vi "运维调试_采配水.vi"() -> ()   [LabVIEW 2016, in "PLC.lvlib"]
uses:
  PLC.lvlib
  <vilib>/Plasmionique/MB Master/MB_Master/MB_Master.lvclass
  <vilib>/Utility/miscctls.llb/LVPointTypeDef.ctl
  <vilib>/Plasmionique/MB Master/MB_Master_Serial/MB_Master_Serial.lvclass
  D:/Program Files (x86)/National Instruments/LabVIEW 2016/vi.lib/Plasmionique/MB Master/MB_Master/MB_Master.lvclass
  <vilib>/Plasmionique/MB Master/MB Master.lvlib
panel:
  out "Y7":bool caption="V6 空压机"
  out "Y6":bool caption="V5 排液阀"
  out "Y5":bool caption="V4 二级清洗阀"
  out "Y4":bool caption="V3 一级清洗阀"
  out "Y3":bool caption="V2 外部管路清洗阀"
  out "Y2":bool caption="M2 增压泵"
  out "Y1":bool caption="V1 进样阀"
  out "Y0":bool caption="M1 潜水泵"
  out "X7":bool caption="采水泵过载检测"
  out "X6":bool caption="断电检测"
  out "X5":bool caption="开门检测"
  out "X4":bool caption="烟雾检测"
  out "X3":bool caption="漏水检测"
  out "X2":bool caption="进样检测"
  out "X1":bool
  out "X0":bool caption="采样池液位开关"
  out "R109":i16 caption="配水时间"
  out "集成报警信息":string
  out "R108":i16 caption="自来水报警"
  out "R107":i16 caption="采水池液位报警设置"
  out "R106":i16 caption="进样超时设置"
  out "R105":i16 caption="二级清洗时间"
  out "R104":i16 caption="一级清洗时间"
  out "R103":i16 caption="外部管路清洗时间"
  out "R102":i16 caption="静置沉淀时间"
  out "R101":i16 caption="内部管路润洗时间"
  out "R100":i16 caption="外部管路润洗时间"
  out "R2":i16
  out "R1":i16
  out "多列列表框":i32(listbox)
  out "R19":i16
  out "R18":i16
  out "R17":i16
  out "R16":i16
  out "R15":i16
  out "R14":i16
  out "R13":i16
  out "R12":i16
  in  "V6":bool
  in  "V5":bool
  in  "V4":bool
  in  "V3":bool
  in  "V2":bool
  in  "M2":bool
  in  "V1":bool
  in  "M1":bool
  in  "返回":bool
  in  "参数设置":bool
  in  "单步启动":bool
  in  "启动":bool
  in  "停止":bool
  # "S"
  # "S"
  # "S"
  # "S"
  # "S"
  # "S"
  # "S"
  # "S"
  # "S"
  # "S"
  # "单步计时："
  # "s"
  # "流程计时："
  # "s"
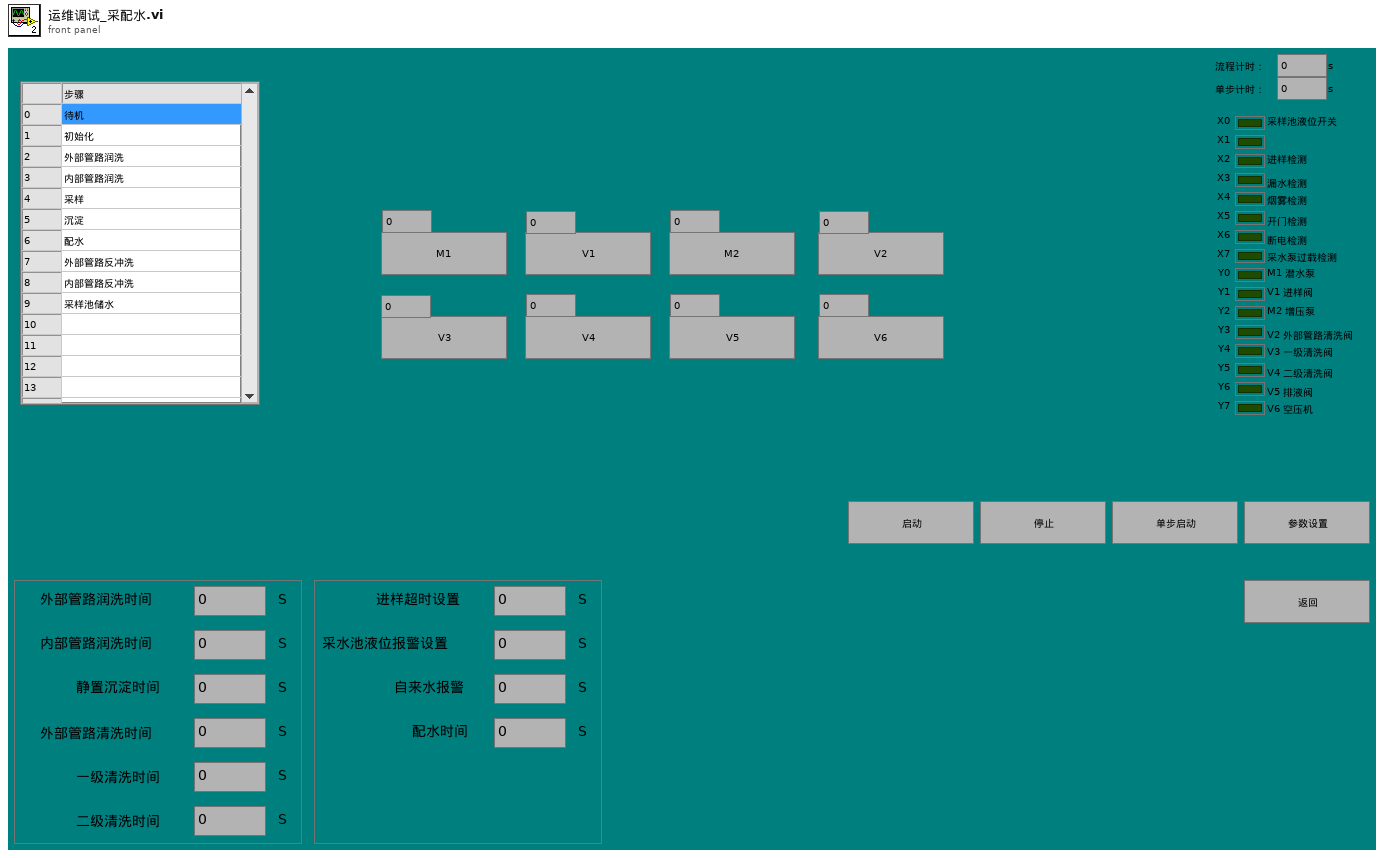
[diagram p1: front panel]
types:
  T1 = typedef "LVPointTypeDef.ctl" = cluster{"Horizontal":i16, "Vertical":i16}
  T2 = cluster{"时间标识":timestamp, "设备":string, "日志信息":string}
  T3 = cluster{"R0":i16, "R1":i16, "R2":i16, "R3":i16, "R4":i16, "R5":i16, "R6":i16, "R7":i16, "R8":i16, "R9":i16, "R10":i16, "R11":i16, "R12":i16, "R13":i16, "R14":i16, "R15":i16, "R16":i16, "R17":i16, "R18":i16, "R19":i16}
  T4 = cluster{"coil values[0]":bool, "coil values[1]":bool, "coil values[2]":bool, "coil values[3]":bool, "coil values[4]":bool, "coil values[5]":bool, "coil values[6]":bool, "coil values[7]":bool, "coil values[8]":bool, "coil values[9]":bool, "coil values[10]":bool, "coil values[11]":bool, "coil values[12]":bool, "coil values[13]":bool, "coil values[14]":bool, "coil values[15]":bool}
  T5 = cluster{"seconds since 1Jan1904":timestamp, "table输入":string, string, "table输入":string}
  T6 = cluster{"时间标识":timestamp, "设备":string, "日志信息":string, "流程参数":string}
  T7 = cluster{"命令":string, cluster{"starting address":u16, "holding register value":u16}}
  T8 = cluster{"命令":string, "数据":cluster{"starting address":u16, "holding register value":u16}}
  T9 = cluster{"命令":string, "数据":cluster{"starting address":u16, "holding register values":u16[]}}
  T10 = cluster{"命令":string, "data":cluster{"starting address":u16, "coil values":bool[]}}
  T11 = enum32{"Bad", "Idle", "Run top level", "Running"}
  T12 = cluster{"baud rate (bps)":u32, "stop bits":u16, "parity":u16, "flow control":u16, "timeout":u32, "retries":i32}
  T13 = cluster{"starting address":u16, "holding register values":u16[]}
  T14 = cluster{"starting address":u16, "holding register value":u16}
  T15 = cluster{"starting address":u16, "coil values":bool[]}
  T16 = cluster{"Registers[0]":u16, "Registers[1]":u16, "Registers[2]":u16, "Registers[3]":u16, "Registers[4]":u16, "Registers[5]":u16, "Registers[6]":u16, "Registers[7]":u16, "Registers[8]":u16, "Registers[9]":u16, "Registers[10]":u16, "Registers[11]":u16, "Registers[12]":u16, "Registers[13]":u16, "Registers[14]":u16, "Registers[15]":u16, "Registers[16]":u16, "Registers[17]":u16, "Registers[18]":u16, "Registers[19]":u16}
  T17 = cluster{"Registers[0]":u16, "Registers[1]":u16, "Registers[2]":u16, "Registers[3]":u16, "Registers[4]":u16, "Registers[5]":u16}
  T18 = cluster{"Coils[0]":bool, "Coils[1]":bool, "Coils[2]":bool, "Coils[3]":bool, "Coils[4]":bool, "Coils[5]":bool, "Coils[6]":bool, "Coils[7]":bool, "Coils[8]":bool, "Coils[9]":bool, "Coils[10]":bool, "Coils[11]":bool, "Coils[12]":bool, "Coils[13]":bool, "Coils[14]":bool, "Coils[15]":bool}
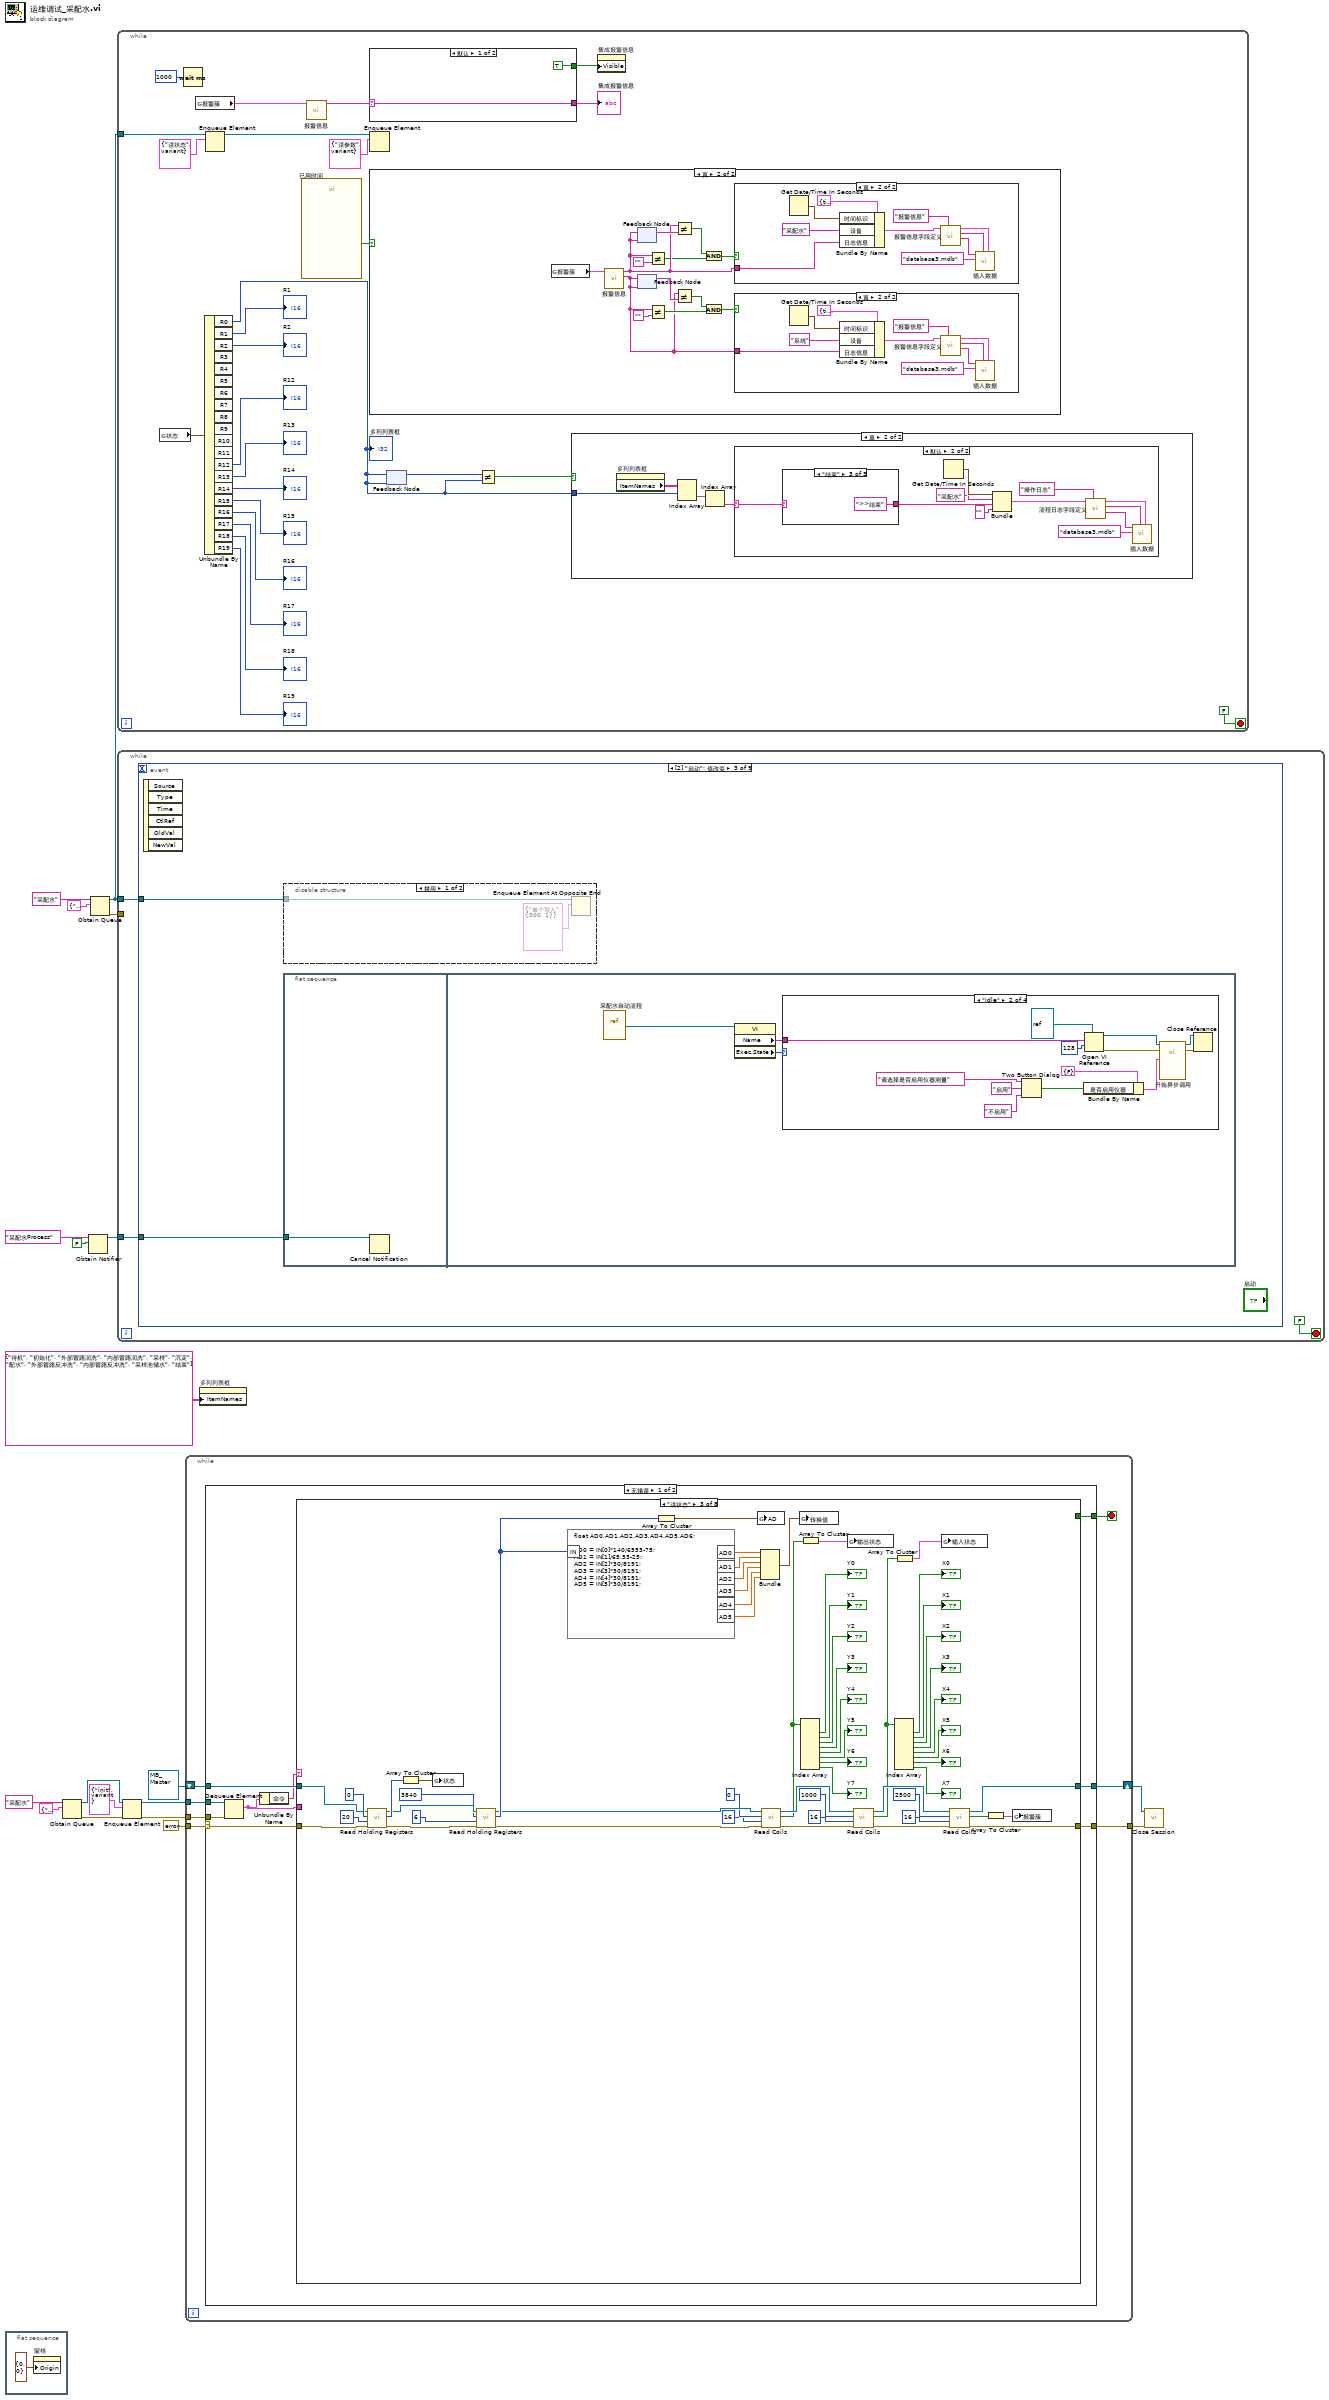
[diagram p0: block diagram]
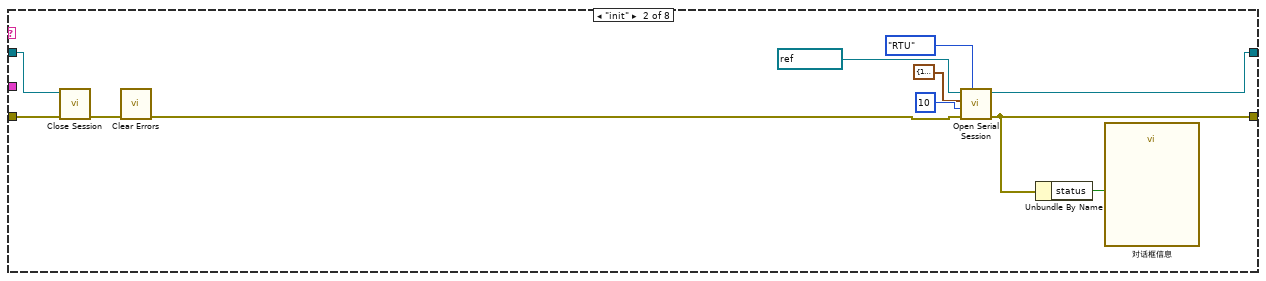
[diagram p3: hidden frame]
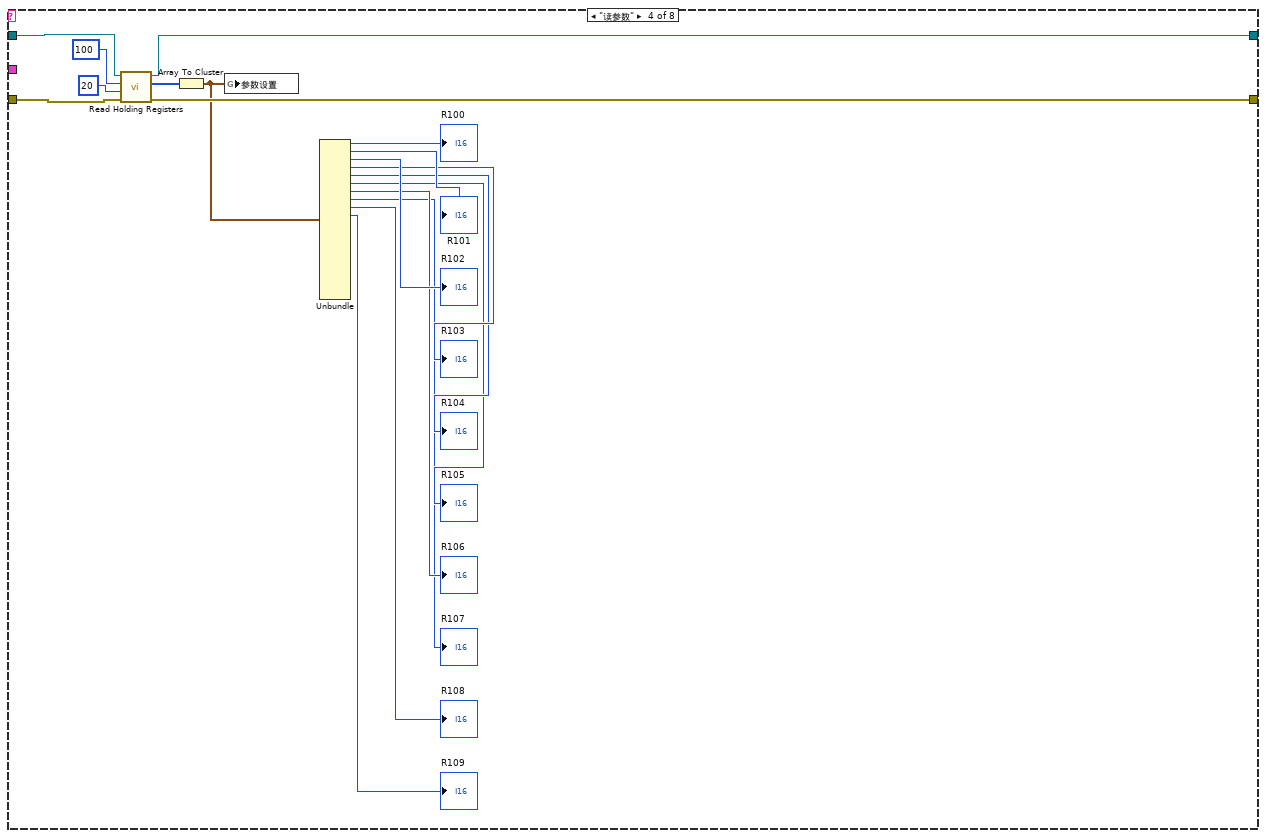
[diagram p4: hidden frame]
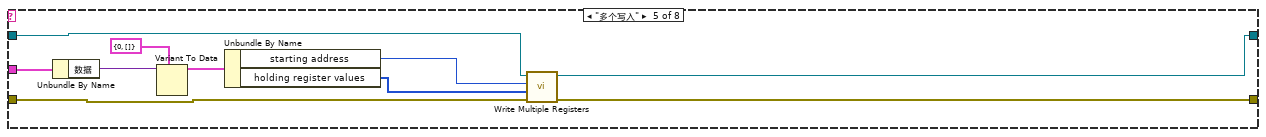
[diagram p5: hidden frame]
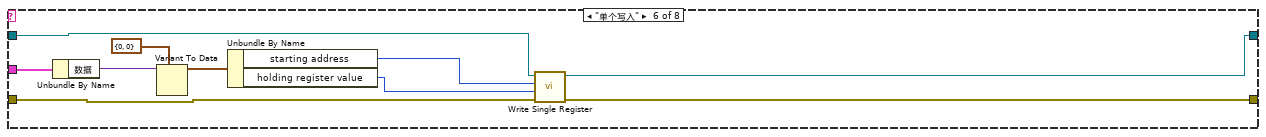
[diagram p6: hidden frame]
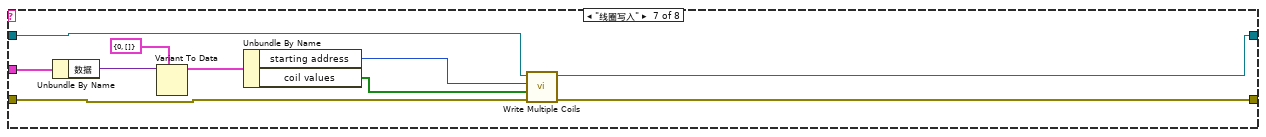
[diagram p7: hidden frame]
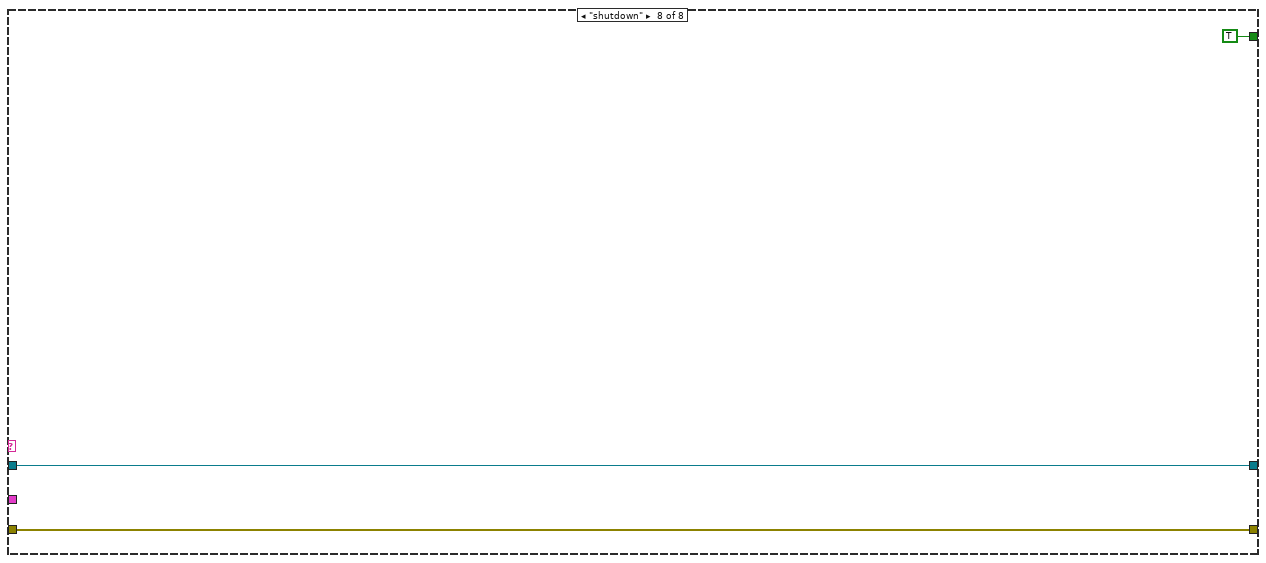
[diagram p8: hidden frame]
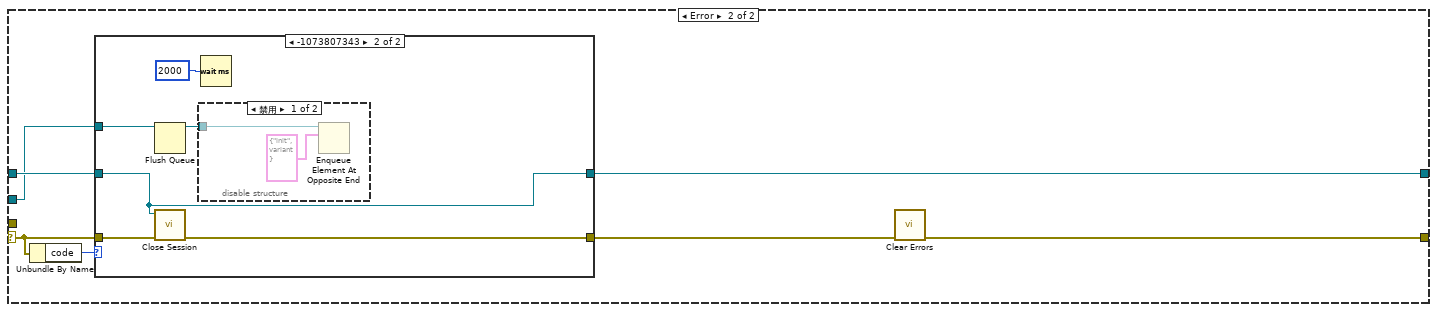
[diagram p9: hidden frame]
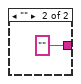
[diagram p15: hidden frame]
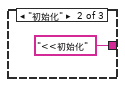
[diagram p19: hidden frame]
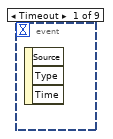
[diagram p20: hidden frame]
diagram:
  n1 = flat-sequence {
    frame #0 {
      n2 = property on="窗格" class="Pane"("Origin"=T1 {"Horizontal"=0, "Vertical"=0} ("原点")) -> ()  [unwired: 2 in, 2 out]
    }
  }
  n3 = Obtain Queue(name (unnamed)="采配水" ("名称（未命名）"), element data type=cluster{"命令":string, "数据":variant} {"命令"="", "数据"=variant}) -> (queue out=w9:refnum<queue>, error out=w8:errorcluster)  [unwired: 3 in, 1 out]
  n4 = Obtain Notifier(name (unnamed)="采配水Process" ("名称（未命名）"), notification data type=FALSE) -> (notifier out=w12:refnum<notifier>)  [unwired: 2 in, 2 out]
  n5 = Obtain Queue(name (unnamed)="采配水" ("名称（未命名）"), element data type=cluster{"命令":string, "数据":variant} {"命令"="", "数据"=variant}) -> (queue out=w16:refnum<queue>, error out=w17:errorcluster)  [unwired: 3 in, 1 out]
  n6 = while {
    tunnel: w16 -> [w44]
    stop <- FALSE stop-if-true
    n7 = global read "采配水全局变量.vi" "状态"() -> (w42:T3)
    n8 = Wait (ms)(milliseconds to wait=u32 1000 ("等待时间（毫秒）")) -> ()  [unwired: 1 out]
    n9 = global read "采配水全局变量.vi" "报警簇"() -> (w30:T4)
    n10 = Unbundle By Name(w42) -> ("R0"=w21:i16, "R1"=→"R1":i16, "R2"=→"R2":i16, "R12"=→"R12":i16, "R13"=→"R13":i16, "R14"=→"R14":i16, "R15"=→"R15":i16, "R16"=→"R16":i16, "R17"=→"R17":i16, "R18"=→"R18":i16, "R19"=→"R19":i16)  [unwired: 9 out]
    "多列列表框" <- w21
    n11 = Enqueue Element(queue=w44, element=cluster{"命令":string, "数据":variant} {"命令"="读状态", "数据"=variant} ("元素")) -> (queue out=w24:refnum<queue>)  [unwired: 2 in, 2 out]
    n12 = call "已用时间"() -> ("Time has Elapsed"=w27:bool)  [unwired: 12 in, 7 out]
    n13 = call "报警信息.vi"("报警簇"=w30) -> ("采配水报警信息"=w23:string)  [unwired: 9 in, 1 out]
    n14 = case shown="默认" w23 {
      selector: w23 -> [w80 _]
      tunnel: [w80 "" ("字符串")] -> w29
      tunnel: [TRUE ("可见") _] -> w28
      frame Default {
      }
      frame "" {
      }
    }
    "集成报警信息" <- w29
    n15 = Enqueue Element(queue=w24, element=cluster{"命令":string, "数据":variant} {"命令"="读参数", "数据"=variant} ("元素")) -> ()  [unwired: 2 in, 3 out]
    n16 = case shown="真" w27 {
      frame False {
      }
      frame True {
        n17 = global read "采配水全局变量.vi" "报警簇"() -> (w58:T4)
        n18 = call "报警信息.vi"("报警簇"=w58) -> ("系统报警信息"=w47:string, "采配水报警信息"=w54:string)  [unwired: 9 in]
        n19 = feedback #1(w54) -> (w57:string)
        n20 = feedback-in #1(w54) -> ()
        n21 = feedback #2(w47) -> (w48:string)
        n22 = feedback-in #2(w47) -> ()
        n23 = Not Equal?(x=w54, y="") -> (x != y?=w52:bool)
        n24 = Not Equal?(x=w47, y="") -> (x != y?=w51:bool)
        n25 = Not Equal?(x=w54, y=w57) -> (x != y?=w56:bool)
        n26 = Not Equal?(x=w47, y=w48) -> (x != y?=w49:bool)
        n27 = And(x=w56, y=w52) -> (x .and. y?=w55:bool)
        n28 = And(x=w49, y=w51) -> (x .and. y?=w46:bool)
        n29 = case shown="真" w55 {
          tunnel: w54 -> [_ w69]
          frame False {
          }
          frame True {
            n30 = Get Date/Time In Seconds() -> (seconds since 1Jan1904=w71:timestamp)
            n31 = Bundle By Name(cluster=T2 {"时间标识"=timestamp(0 s since 1904-01-01), "设备"="", "日志信息"=""} ("data in"), "时间标识"=w71, "设备"="采配水", "日志信息"=w69) -> (w72:T2)
            n32 = call "报警信息字段定义.vi"("table输入"="报警信息", "data in"=w72) -> ("table输出"=w76:string, "columns"=w77:string[], "data out"=w78:T2)  [unwired: 7 in]
            n33 = call "插入数据.vi"("data"=w78, "columns"=w77, "database"="database3.mdb", "table"=w76) -> ()  [unwired: 7 in, 1 out]
          }
        }
        n34 = case shown="真" w46 {
          tunnel: w47 -> [_ w59]
          frame False {
          }
          frame True {
            n35 = Get Date/Time In Seconds() -> (seconds since 1Jan1904=w61:timestamp)
            n36 = Bundle By Name(cluster=T2 {"时间标识"=timestamp(0 s since 1904-01-01), "设备"="", "日志信息"=""} ("data in"), "时间标识"=w61, "设备"="系统", "日志信息"=w59) -> (w62:T2)
            n37 = call "报警信息字段定义.vi"("table输入"="报警信息", "data in"=w62) -> ("table输出"=w66:string, "columns"=w67:string[], "data out"=w68:T2)  [unwired: 7 in]
            n38 = call "插入数据.vi"("data"=w68, "columns"=w67, "database"="database3.mdb", "table"=w66) -> ()  [unwired: 7 in, 1 out]
          }
        }
      }
    }
    n39 = feedback-in #3(w21) -> ()
    n40 = feedback #3(w21) -> (w22:i16)
    n41 = Not Equal?(x=w22, y=w21) -> (x != y?=w31:bool)
    n42 = case shown="真" w31 {
      tunnel: w21 -> [_ w84]
      frame False {
      }
      frame True {
        n43 = property on="多列列表框" class="MCListbox (严格)"() -> ("ItemNames"=w85:string[][])  [unwired: 2 in, 2 out]
        n44 = Index Array(array=w85, index (row)=w84) -> (element=w83:string[])  [unwired: 1 in]
        n45 = Index Array(array=w83) -> (element=w82:string)  [unwired: 1 in]
        n46 = case shown="默认" w82 {
          selector: w82 -> [_ w87]
          frame "待机" {
          }
          frame Default {
            n47 = case shown="\"结束\"" w87 {
              selector: w87 -> [w97 _ _]
              tunnel: [w97 "<<初始化" ">>结束"] -> w86
              frame Default {
              }
              frame "初始化" {
              }
              frame "结束" {
              }
            }
            n48 = Get Date/Time In Seconds() -> (seconds since 1Jan1904=w91:timestamp)
            n49 = Bundle("seconds since 1Jan1904"=w91, "table输入"="采配水", w86, "table输入"="") -> (w89:T5)  [unwired: 1 in]
            n50 = call "流程日志字段定义.vi"("table输入"="操作日志", "data in"=w89) -> ("table输出"=w94:string, "columns"=w95:string[], "data out"=w96:T6)  [unwired: 7 in]
            n51 = call "插入数据.vi"("data"=w96, "columns"=w95, "database"="database3.mdb", "table"=w94) -> ()  [unwired: 7 in, 1 out]
          }
        }
      }
    }
    n52 = property on="集成报警信息" class="Str"("Visible"=w28) -> ()  [unwired: 2 in, 2 out]
  }
  n53 = while {
    tunnel: w16 -> [w101]
    tunnel: w17 -> [_]
    tunnel: w12 -> [w100]
    stop <- FALSE stop-if-true
    n54 = event shown="[2] \"启动\": 值改变" {
      selector: _ -> [_ _ _ _ _ _ _ _ _]
      dyn-events: _ -> [_ _ _ _ _ _ _ _ _]
      timeout: _ -> [_ _ _ _ _ _ _ _ _]
      tunnel: w101 -> [_ w105 w108 w132 w147 _ _ _ w165]
      tunnel: w100 -> [_ w104 w107 _ _ _ _ _ _]
      event Timeout {
        n55 = event-data() -> ()  [unwired: 1 in, 3 out]
      }
      event "停止": Value Change {
        n56 = event-data() -> ()  [unwired: 1 in, 6 out]
        n57 = Send Notification(notification=TRUE ("通知"), notifier=w104) -> ()  [unwired: 1 in, 2 out]
        n58 = Enqueue Element At Opposite End(queue=w105, element=T7 {"命令"="单个写入", {"starting address"=300, "holding register value"=2}} ("元素")) -> ()  [unwired: 2 in, 3 out]
      }
      event "启动": Value Change {
        n59 = event-data() -> ()  [unwired: 1 in, 6 out]
        n60 = disable-structure shown="禁用" {
          disable-tunnel: w108 -> [w128 _]
          frame Disabled {
            n61 = Enqueue Element At Opposite End(queue=w128, element=T7 {"命令"="单个写入", {"starting address"=300, "holding register value"=1}} ("元素")) -> ()  [unwired: 2 in, 3 out]
          }
          frame Enabled {
          }
        }
        n62 = flat-sequence {
          tunnel: w107 -> [w109]
          frame #0 {
            n63 = Cancel Notification(0:w109) -> ()  [unwired: 1 in, 3 out]
          }
          frame #1 {
            n64 = vi-ref "采配水自动流程.vi"() -> (w112:refnum<vi>)
            n65 = property class="VI"(reference=w112) -> ("Name"=w111:string, "Exec.State"=w110:T11)  [unwired: 1 in, 2 out]
            n66 = case shown="\"Idle\"" w110 {
              tunnel: w111 -> [_ w125 _ _]
              frame "Bad", Default {
              }
              frame "Idle" {
                n67 = Two Button Dialog(message="请选择是否启用仪器测量" ("消息"), 1:"不启用" ("F按钮名称（“取消”）"), 2:"启用" ("T按钮名称（“确定”）")) -> (T button?=w115:bool)
                n68 = Bundle By Name(cluster=cluster{"是否启用仪器":bool} {"是否启用仪器"=FALSE} ("参数"), "是否启用仪器"=w115) -> (w113:cluster{"是否启用仪器":bool})
                n69 = Open VI Reference(type specifier VI Refnum (for type only)=refnum<vi> refnum, vi path=w125, options=128 ("选项")) -> (vi reference=w123:refnum<vi>, error out=w120:errorcluster)  [unwired: 3 in]
                n70 = call-by-ref "开始异步调用"(reference=w123, error in=w120, "参数"=w113) -> (reference out=w121:refnum<vi>, error out=w119:errorcluster)  [unwired: 11 in]
                n71 = Close Reference(reference=w121, error in (no error)=w119) -> ()  [unwired: 1 out]
              }
              frame "Run top level" {
              }
              frame "Running" {
                n72 = One Button Dialog(message="流程已经运行,无须重复启动" ("消息")) -> ()  [unwired: 1 in, 1 out]
              }
            }
          }
        }
      }
      event "单步启动": Value Change {
        n73 = event-data() -> ()  [unwired: 1 in, 6 out]
        n74 = call "单步启动对话框.vi"() -> ("单步启动步骤输出"=w129:u16)  [unwired: 11 in]
        n75 = Bundle By Name(cluster=T8 {"命令"="单个写入", "数据"={"starting address"=301, "holding register value"=0}} ("元素"), "数据.holding register value"=w129) -> (w130:T8)
        n76 = Enqueue Element At Opposite End(queue=w132, element=w130) -> ()  [unwired: 2 in, 3 out]
      }
      event "R100", "R101", "R102", "R103", "R104", "R105", "R106", "R107", "R108", "R109": Value Change {
        n77 = event-data() -> ()  [unwired: 1 in, 6 out]
        n78 = local read "R100"() -> (w142:i16)
        n79 = local read "R101"() -> (w141:i16)
        n80 = local read "R102"() -> (w140:i16)
        n81 = local read "R103"() -> (w139:i16)
        n82 = local read "R104"() -> (w138:i16)
        n83 = local read "R105"() -> (w137:i16)
        n84 = local read "R106"() -> (w136:i16)
        n85 = local read "R107"() -> (w135:i16)
        n86 = local read "R108"() -> (w134:i16)
        n87 = local read "R109"() -> (w133:i16)
        n88 = Build Array(w142, w141, w140, w139, w138, w137, w136, w135, w134, w133) -> (w143:i16[])
        n89 = Bundle By Name(cluster=T9 {"命令"="多个写入", "数据"={"starting address"=0, "holding register values"=[]}} ("元素"), "数据.starting address"=u16 100, "数据.holding register values"=w143) -> (w144:T9)
        n90 = Enqueue Element At Opposite End(queue=w147, element=w144) -> ()  [unwired: 2 in, 3 out]
      }
      event "R100", "R101", "R102", "R103", "R104", "R105", "R106", "R107", "R108", "R109": Mouse Down {
        n91 = event-data() -> ("CtlRef"=w151:refnum<vi>)  [unwired: 1 in, 7 out]
        n92 = property class="DigNum (严格)"(reference=w151) -> (reference out=w149:refnum<vi>, "Value"=w150:i16)  [unwired: 1 in, 1 out]
        n93 = call "数字键盘.vi"("OldNumber"=w150) -> ("NewNumber"=w148:sgl)
        n94 = property class="DigNum (严格)"(reference=w149, "Val(Sgnl)"=w148) -> ()  [unwired: 1 in, 2 out]
      }
      event "参数设置": Value Change {
        n95 = event-data() -> ()  [unwired: 1 in, 6 out]
        n96 = property on="窗格" class="Pane"("Origin"=T1 {"Horizontal"=0, "Vertical"=528} ("原点")) -> ()  [unwired: 2 in, 2 out]
      }
      event "返回": Value Change {
        n97 = event-data() -> ()  [unwired: 1 in, 6 out]
        n98 = property on="窗格" class="Pane"("Origin"=T1 {"Horizontal"=0, "Vertical"=0} ("原点")) -> ()  [unwired: 2 in, 2 out]
      }
      event "M1", "V1", "M2", "V2", "V3", "V4", "V5", "V6": Value Change {
        n99 = event-data() -> ()  [unwired: 1 in, 6 out]
        n100 = Build Array("M1", "V1", "M2", "V2", "V3", "V4", "V5", "V6") -> (w154:bool[])
        n101 = Bundle By Name(cluster=T10 {"命令"="线圈写入", "data"={"starting address"=2400, "coil values"=[]}} ("元素"), "data.coil values"=w154) -> (w155:T10)
        n102 = Enqueue Element(queue=w165, element=w155) -> ()  [unwired: 2 in, 3 out]
      }
    }
  }
  n103 = Enqueue Element(queue=w9, element=cluster{"命令":string, "数据":variant} {"命令"="init", "数据"=variant} ("元素"), error in (no error)=w8) -> (queue out=w4:refnum<queue>, error out=w6:errorcluster)  [unwired: 1 in, 1 out]
  n104 = while {
    tunnel: w4 -> [w168]
    tunnel: w6 -> [w167]
    shift-right: [w172] -> w1
    shift-left: refnum<class "MB_Master.lvclass"> refnum ("MB session in") -> [w171]
    tunnel: errorcluster {"status"=FALSE, "code"=0, "source"=""} ("error out") -> [w169]
    tunnel: [w170] -> w2
    stop <- w166 stop-if-true
    n105 = case shown="无错误" w169 {
      selector: w169 -> [w178 w305]
      tunnel: [w181 w304] -> w172
      tunnel: w171 -> [w180 w306]
      tunnel: [w179 w302] -> w170
      tunnel: w168 -> [w175 w301]
      tunnel: w167 -> [w174 _]
      tunnel: [w176 _] -> w166
      frame No Error {
        n106 = Dequeue Element(queue=w175, error in (no error)=w174) -> (element=w173:cluster{"命令":string, "数据":variant})  [unwired: 1 in, 3 out]
        n107 = Unbundle By Name(w173) -> ("命令"=w177:string)
        n108 = case shown="\"读状态\"" w177 {
          tunnel: [w183 w187 w214 w262 w274 w284 w294 w299] -> w181
          tunnel: w180 -> [w183 w191 w234 w267 w277 w287 w297 w299]
          tunnel: [w182 w189 w213 w261 w275 w285 w295 w298] -> w179
          tunnel: w178 -> [w182 w193 w237 w266 w276 w286 w296 w298]
          tunnel: [_ _ _ _ _ _ _ TRUE] -> w176
          tunnel: w173 -> [_ _ _ _ w273 w283 w293 _]
          frame "idle", Default {
          }
          frame "init" {
            n109 = call-dynamic "Close Session.vi"("error in (no error)"=w193, "MB session in"=w191) -> ("error out"=w192:errorcluster)  [unwired: 9 in]
            n110 = call <vilib>:"Clear Errors.vi"("error in (no error)"=w192) -> ("error out"=w190:errorcluster)  [unwired: 5 in, 1 out]
            n111 = call <vilib>:"Open Serial Session.vi"("Mode (RTU)"=enum16{"RTU", "ASCII"}."RTU", "Error in"=w190, "Slave ID"=u8 10, "Serial Config"=T12 {"baud rate (bps)"=115200, "stop bits"=10, "parity"=0, "flow control"=0, "timeout"=1000, "retries"=1}, "VISA Resource"=refnum<visa-resource-name> "COM2" ("VISA resource name")) -> ("Error out"=w189:errorcluster, "MB_Serial session"=w187:refnum<class "MB_Master_Serial.lvclass">)  [unwired: 5 in]
            n112 = Unbundle By Name(w189) -> ("status"=w194:bool)
            n113 = call "对话框信息"("Enable"=w194) -> ()  [unwired: 9 in, 2 out]
          }
          frame "读状态" {
            n114 = call <vilib>:"Read Holding Registers.vi"("error in (no error)"=w237, "quantity"=u16 20 ("number of holding registers"), "starting address"=u16 0, "MB session in"=w234) -> ("error out"=w230:errorcluster, "Registers"=w233:u16[], "MB session out"=w232:refnum<class "MB_Master.lvclass">)  [unwired: 5 in]
            n115 = Array To Cluster(array=w233) -> (cluster=w239:T16)
            n116 = global write "采配水全局变量.vi" "状态"(w239) -> ()
            n117 = call <vilib>:"Read Holding Registers.vi"("error in (no error)"=w230, "quantity"=u16 6 ("number of holding registers"), "starting address"=u16 3840, "MB session in"=w232) -> ("error out"=w226:errorcluster, "Registers"=w231:u16[], "MB session out"=w227:refnum<class "MB_Master.lvclass">)  [unwired: 5 in]
            n118 = formula code="float AD0,AD1,AD2,AD3,AD4,AD5,AD6;\n\nAD0 = IN[0]*140/6553-75;\nAD1 = IN[1]/65.53-25;\nAD2 = IN[2]*30/8191;\nAD3 = IN[3]*30/8191;\nAD4 = IN[4]*30/8191;\nAD5 = IN[5]*30/8191;"("IN"=w231) -> ("AD0"=w245:dbl, "AD1"=w244:dbl, "AD2"=w243:dbl, "AD3"=w242:dbl, "AD4"=w241:dbl, "AD5"=w240:dbl)
            n119 = Array To Cluster(array=w231) -> (cluster=w247:T17)
            n120 = global write "采配水全局变量.vi" "AD"(w247) -> ()
            n121 = Bundle(w245, w244, w243, w242, w241, w240) -> (w246:cluster{dbl, dbl, dbl, dbl, dbl, dbl})  [unwired: 1 in]
            n122 = call <vilib>:"Read Coils.vi"("error in (no error)"=w226, "quantity"=u16 16 ("number of coils"), "starting address"=u16 0, "MB session in"=w227) -> ("error out"=w222:errorcluster, "Coils"=w203:bool[], "MB session out"=w223:refnum<class "MB_Master.lvclass">)  [unwired: 5 in]
            n123 = global write "采配水全局变量.vi" "转换值"(w246) -> ()
            n124 = Index Array(array=w203) -> (element #1=→"Y0":bool, element #2=→"Y1":bool, element #3=→"Y2":bool, element #4=→"Y3":bool, element #5=→"Y4":bool, element #6=→"Y5":bool, element #7=→"Y6":bool, element #8=→"Y7":bool)  [unwired: 8 in]
            n125 = Array To Cluster(array=w203) -> (cluster=w248:T18)
            n126 = global write "采配水全局变量.vi" "输出状态"(w248) -> ()
            n127 = call <vilib>:"Read Coils.vi"("error in (no error)"=w222, "quantity"=u16 16 ("number of coils"), "starting address"=u16 1000, "MB session in"=w223) -> ("error out"=w218:errorcluster, "Coils"=w212:bool[], "MB session out"=w219:refnum<class "MB_Master.lvclass">)  [unwired: 5 in]
            n128 = Index Array(array=w212) -> (element #1=→"X0":bool, element #2=→"X1":bool, element #3=→"X2":bool, element #4=→"X3":bool, element #5=→"X4":bool, element #6=→"X5":bool, element #7=→"X6":bool, element #8=→"X7":bool)  [unwired: 8 in]
            n129 = Array To Cluster(array=w212) -> (cluster=w249:T18)
            n130 = global write "采配水全局变量.vi" "输入状态"(w249) -> ()
            n131 = call <vilib>:"Read Coils.vi"("error in (no error)"=w218, "quantity"=u16 16 ("number of coils"), "starting address"=u16 2500, "MB session in"=w219) -> ("error out"=w213:errorcluster, "Coils"=w215:bool[], "MB session out"=w214:refnum<class "MB_Master.lvclass">)  [unwired: 5 in]
            n132 = Array To Cluster(array=w215) -> (cluster=w238:T18)
            n133 = global write "采配水全局变量.vi" "报警簇"(w238) -> ()
          }
          frame "读参数" {
            n134 = call <vilib>:"Read Holding Registers.vi"("error in (no error)"=w266, "quantity"=u16 20 ("number of holding registers"), "starting address"=u16 100, "MB session in"=w267) -> ("error out"=w261:errorcluster, "Registers"=w263:u16[], "MB session out"=w262:refnum<class "MB_Master.lvclass">)  [unwired: 5 in]
            n135 = Array To Cluster(array=w263) -> (cluster=w250:T16)
            n136 = global write "采配水全局变量.vi" "参数设置"(w250) -> ()
            n137 = Unbundle(w250) -> ("Registers[0]"=→"R100":u16, "Registers[1]"=→"R101":u16, "Registers[2]"=→"R102":u16, "Registers[3]"=→"R103":u16, "Registers[4]"=→"R104":u16, "Registers[5]"=→"R105":u16, "Registers[6]"=→"R106":u16, "Registers[7]"=→"R107":u16, "Registers[8]"=→"R108":u16, "Registers[9]"=→"R109":u16)  [unwired: 10 out]
          }
          frame "多个写入" {
            n138 = Unbundle By Name(w273) -> ("数据"=w272:variant)
            n139 = Variant To Data(type=T13 {"starting address"=0, "holding register values"=[]}, Variant=w272) -> (data=w270:T13)  [unwired: 1 in, 1 out]
            n140 = Unbundle By Name(w270) -> ("starting address"=w269:u16, "holding register values"=w268:u16[])
            n141 = call <vilib>:"Write Multiple Registers.vi"("error in (no error)"=w276, "values"=w268, "starting address"=w269, "MB session in"=w277) -> ("error out"=w275:errorcluster, "MB session out"=w274:refnum<class "MB_Master.lvclass">)  [unwired: 6 in]
          }
          frame "单个写入" {
            n142 = Unbundle By Name(w283) -> ("数据"=w282:variant)
            n143 = Variant To Data(type=T14 {"starting address"=0, "holding register value"=0}, Variant=w282) -> (data=w280:T14)  [unwired: 1 in, 1 out]
            n144 = Unbundle By Name(w280) -> ("starting address"=w279:u16, "holding register value"=w278:u16)
            n145 = call <vilib>:"Write Single Register.vi"("error in (no error)"=w286, "value"=w278, "address"=w279, "MB session in"=w287) -> ("error out"=w285:errorcluster, "MB session out"=w284:refnum<class "MB_Master.lvclass">)  [unwired: 6 in]
          }
          frame "线圈写入" {
            n146 = Unbundle By Name(w293) -> ("数据"=w292:variant)
            n147 = Variant To Data(type=T15 {"starting address"=0, "coil values"=[]}, Variant=w292) -> (data=w290:T15)  [unwired: 1 in, 1 out]
            n148 = Unbundle By Name(w290) -> ("starting address"=w289:u16, "coil values"=w288:bool[])
            n149 = call <vilib>:"Write Multiple Coils.vi"("error in (no error)"=w296, "values"=w288, "starting address"=w289, "MB session in"=w297) -> ("error out"=w295:errorcluster, "MB session out"=w294:refnum<class "MB_Master.lvclass">)  [unwired: 6 in]
          }
          frame "shutdown" {
          }
        }
      }
      frame Error {
        n150 = Unbundle By Name(w305) -> ("code"=w307:i32)
        n151 = case shown="-1073807343" w307 {
          tunnel: w306 -> [w309 w313]
          tunnel: w305 -> [w308 w315]
          tunnel: [w308 w314] -> w303
          tunnel: [w309 w313] -> w304
          tunnel: w301 -> [_ w312]
          frame Default {
          }
          frame -1073807343 {
            n152 = Flush Queue(queue=w312) -> (queue out=w311:refnum<queue>)  [unwired: 1 in, 2 out]
            n153 = call-dynamic "Close Session.vi"("error in (no error)"=w315, "MB session in"=w313) -> ("error out"=w314:errorcluster)  [unwired: 9 in]
            n154 = disable-structure shown="禁用" {
              disable-tunnel: w311 -> [w316 _]
              frame Disabled {
                n155 = Enqueue Element At Opposite End(queue=w316, element=cluster{"命令":string, "数据":variant} {"命令"="init", "数据"=variant} ("元素")) -> ()  [unwired: 2 in, 3 out]
              }
              frame Enabled {
              }
            }
            n156 = Wait (ms)(milliseconds to wait=u32 2000 ("等待时间（毫秒）")) -> ()  [unwired: 1 out]
          }
        }
        n157 = call <vilib>:"Clear Errors.vi"("error in (no error)"=w303) -> ("error out"=w302:errorcluster)  [unwired: 5 in, 1 out]
      }
    }
  }
  n158 = property on="多列列表框" class="MCListbox (严格)"("ItemNames"=string[][] [["待机"], ["初始化"], ["外部管路润洗"], ["内部管路润洗"], ["采样"], ["沉淀"], ["配水"], ["外部管路反冲洗"], ["内部管路反冲洗"], ["采样池储水"], ["结束"]] ("项名")) -> ()  [unwired: 2 in, 2 out]
  n159 = call-dynamic "Close Session.vi"("error in (no error)"=w2, "MB session in"=w1) -> ()  [unwired: 9 in, 1 out]
